vi "Spectrometer_R&S.vi"(11 "position_xyz":T2 {"Position Z" min=0.0 max=10.0 step=0.001 format="%.3f"; "Position Y" min=-10.0 max=10.0 step=0.1 format="%.3f"; "Position X" min=-10.0 max=10.0 step=0.1 format="%.3f"}) -> ()   [LabVIEW 2014]
uses:
  <vilib>/DAQmx/write.llb/DAQmx Write (Digital Bool 1Line 1Point).vi
  <vilib>/Analysis/baseanly.llb/Vector x A.vi
  GLOBAL_VAR.vi
  <vilib>/DAQmx/miscellaneous.llb/DAQmx Fill In Error Info.vi
  <vilib>/Analysis/Matrix/Numeric/Conversions/Array To Matrix - RA2.vi
  <vilib>/DAQmx/create/channels.llb/DAQmx Create Channel (CO-Pulse Generation-Ticks).vi
  <vilib>/DAQmx/create/channels.llb/DAQmx Create Channel (DO-Digital Output).vi
  <vilib>/DAQmx/configure/trigger.llb/DAQmx Start Trigger (Digital Edge).vi
  <resource>/objmgr/daqmx.rc
  <vilib>/Analysis/NI_AALBase.lvlib
  <vilib>/Analysis/Matrix/NI_Matrix.lvlib
  <instrlib>/Rohde&Schwarz RF Signal Generator/Rohde&Schwarz RF Signal Generator.lvlib
panel:
  in  "sweep_parameters":T1={"Repetitions"=1, "Power dBm"=5.999999061226845, "Freq Start [Hz]"=2800000000.0, "Freq Stop [Hz]"=3000000000.0, "Step size [Hz]"=2500000.0, "Dwell Time [ms]"=0.09999999974525053} {"Dwell Time [ms]" min=9.999999747378752e-05 max=4290.0 step=9.999999974752427e-07 format="%.3f"; "Step size [Hz]" min=10000.0 max=20000000000.0 step=1.0 format="%.2p"; "Freq Stop [Hz]" min=10000.0 max=20000000000.0 step=10000.0 format="%.2p"; "Freq Start [Hz]" min=10000.0 max=20000000000.0 step=10000.0 format="%.2p"; "Power dBm" min=-36.0 max=27.0 step=0.009999999776482582 format="%.2f"; "Repetitions" min=1 max=1000 step=1}
  out "File name":string
  in  "Save":bool
  in  "Stop":bool
  out "Run":i32=100
  out "Remain":i32
  out "Intensity Graph":ext[][](graph)
  out "Histogram":cluster{ext[], ext[]}[](graph)=[{[2700000000.0, 2702500000.0, 2705000000.0, 2707500000.0, 2710000000.0, 2712500000.0, 2715000000.0, 2717500000.0, 2720000000.0, 2722500000.0, 2725000000.0, 2727500000.0, 2730000000.0, 2732500000.0, 2735000000.0, 2737500000.0, 2740000000.0, 2742500000.0, 2745000000.0, 2747500000.0, 2750000000.0, 2752500000.0, 2755000000.0, 2757500000.0, 2760000000.0, 2762500000.0, 2765000000.0, 2767500000.0, 2770000000.0, 2772500000.0, 2775000000.0, 2777500000.0, 2780000000.0, 2782500000.0, 2785000000.0, 2787500000.0, 2790000000.0, 2792500000.0, 2795000000.0, 2797500000.0, 2800000000.0, 2802500000.0, 2805000000.0, 2807500000.0, 2810000000.0, 2812500000.0, 2815000000.0, 2817500000.0, 2820000000.0, 2822500000.0, 2825000000.0, 2827500000.0, 2830000000.0, 2832500000.0, 2835000000.0, 2837500000.0, 2840000000.0, 2842500000.0, 2845000000.0, 2847500000.0, 2850000000.0, 2852500000.0, 2855000000.0, 2857500000.0, 2860000000.0, 2862500000.0, 2865000000.0, 2867500000.0, 2870000000.0, 2872500000.0, 2875000000.0, 2877500000.0, 2880000000.0, 2882500000.0, 2885000000.0, 2887500000.0, 2890000000.0, 2892500000.0, 2895000000.0, 2897500000.0, 2900000000.0, 2902500000.0, 2905000000.0, 2907500000.0, 2910000000.0, 2912500000.0, 2915000000.0, 2917500000.0, 2920000000.0, 2922500000.0, 2925000000.0, 2927500000.0, 2930000000.0, 2932500000.0, 2935000000.0, 2937500000.0, 2940000000.0, 2942500000.0, 2945000000.0, 2947500000.0, 2950000000.0, 2952500000.0, 2955000000.0, 2957500000.0, 2960000000.0, 2962500000.0, 2965000000.0, 2967500000.0, 2970000000.0, 2972500000.0, 2975000000.0, 2977500000.0, 2980000000.0, 2982500000.0, 2985000000.0, 2987500000.0, 2990000000.0, 2992500000.0, 2995000000.0, 2997500000.0, 3000000000.0], [26841.121559672197128, 27464.174520667373477, 27576.32405364650522, 29408.099758972323686, 27638.629349746022854, 27576.32405364650522, 27638.629349746022854, 27651.09040896592638, 28398.753962160138, 28311.526547620813311, 28236.76019230139215, 27912.772652583900449, 27850.467356484382814, 27875.389474924189868, 28174.454896201874515, 28697.819383437822648, 28685.35832421791912, 28535.825613579076798, 28809.968916416954391, 29046.729041595121403, 28647.975146558208541, 28523.36455435917327, 28062.305363222742772, 28174.454896201874515, 28473.520317479559163, 27738.31782350525107, 28423.676080599945054, 29133.956456134446093, 28859.8131532965685, 27638.629349746022854, 29133.956456134446093, 27763.239941945058124, 27352.024987688241733, 27439.252402227566423, 28822.429975636857918, 27526.479816766891112, 28548.286672798980325, 27838.006297264479286, 28847.352094076664972, 28884.735271736375553, 29271.02810755338489, 28884.735271736375553, 27289.7196915887241, 28971.962686275700243, 28336.448666060620365, 28548.286672798980325, 27975.077948683418082, 27763.239941945058124, 29470.405055071841321, 28822.429975636857918, 28087.227481662549826, 28286.604429181006259, 27352.024987688241733, 27401.869224567855841, 28398.753962160138, 29308.411285213095471, 28485.98137669946269, 28585.669850458690906, 28710.280442657726175, 28236.76019230139215, 28311.526547620813311, 27576.32405364650522, 27302.180750808627625, 28299.065488400909786, 26878.504737331907709, 28809.968916416954391, 29420.560818192227213, 28859.8131532965685, 27750.778882725154597, 28535.825613579076798, 28398.753962160138, 28261.682310741199204, 28947.040567835893189, 28361.370784500427419, 28785.046797977147337, 28610.59196889849796, 27476.635579887277004, 28062.305363222742772, 28311.526547620813311, 28809.968916416954391, 28647.975146558208541, 28112.14960010235688, 28822.429975636857918, 27738.31782350525107, 28199.377014641681569, 28510.903495139269744, 27451.71346144746995, 28074.766422442646299, 27725.856764285347543, 28635.514087338305014, 28834.891034856761445, 27376.947106128048787, 29096.573278474735512, 28274.143369961102731, 29034.267982375217876, 28560.747732018883852, 27277.258632368820573, 28884.735271736375553, 28049.844304002839245, 27975.077948683418082, 26965.732151871232396, 28809.968916416954391, 28000.000067123225136, 27127.725921729978248, 28037.383244782935718, 28000.000067123225136, 27277.258632368820573, 27800.623119604768705, 28087.227481662549826, 27501.557698327084058, 26778.816263572679492, 26429.906605415380737, 27526.479816766891112, 26442.367664635284264, 26479.750842294994845, 27775.701001164961651, 27040.498507190653559, 26429.906605415380737, 27750.778882725154597, 27464.174520667373477, 27925.233711803803976]}, {[2700000000.0, 2702500000.0, 2705000000.0, 2707500000.0, 2710000000.0, 2712500000.0, 2715000000.0, 2717500000.0, 2720000000.0, 2722500000.0, 2725000000.0, 2727500000.0, 2730000000.0, 2732500000.0, 2735000000.0, 2737500000.0, 2740000000.0, 2742500000.0, 2745000000.0, 2747500000.0, 2750000000.0, 2752500000.0, 2755000000.0, 2757500000.0, 2760000000.0, 2762500000.0, 2765000000.0, 2767500000.0, 2770000000.0, 2772500000.0, 2775000000.0, 2777500000.0, 2780000000.0, 2782500000.0, 2785000000.0, 2787500000.0, 2790000000.0, 2792500000.0, 2795000000.0, 2797500000.0, 2800000000.0, 2802500000.0, 2805000000.0, 2807500000.0, 2810000000.0, 2812500000.0, 2815000000.0, 2817500000.0, 2820000000.0, 2822500000.0, 2825000000.0, 2827500000.0, 2830000000.0, 2832500000.0, 2835000000.0, 2837500000.0, 2840000000.0, 2842500000.0, 2845000000.0, 2847500000.0, 2850000000.0, 2852500000.0, 2855000000.0, 2857500000.0, 2860000000.0, 2862500000.0, 2865000000.0, 2867500000.0, 2870000000.0, 2872500000.0, 2875000000.0, 2877500000.0, 2880000000.0, 2882500000.0, 2885000000.0, 2887500000.0, 2890000000.0, 2892500000.0, 2895000000.0, 2897500000.0, 2900000000.0, 2902500000.0, 2905000000.0, 2907500000.0, 2910000000.0, 2912500000.0, 2915000000.0, 2917500000.0, 2920000000.0, 2922500000.0, 2925000000.0, 2927500000.0, 2930000000.0, 2932500000.0, 2935000000.0, 2937500000.0, 2940000000.0, 2942500000.0, 2945000000.0, 2947500000.0, 2950000000.0, 2952500000.0, 2955000000.0, 2957500000.0, 2960000000.0, 2962500000.0, 2965000000.0, 2967500000.0, 2970000000.0, 2972500000.0, 2975000000.0, 2977500000.0, 2980000000.0, 2982500000.0, 2985000000.0, 2987500000.0, 2990000000.0, 2992500000.0, 2995000000.0, 2997500000.0, 3000000000.0], [27662.305362263847, 27614.704116043806, 27558.75396014644, 27479.62623410005, 27635.264863756656, 27635.514084941045, 27523.73838373851, 27614.704116043802, 27583.17763621744, 27571.58885114293, 27593.520315369973, 27605.109100444486, 27505.545237277456, 27540.685424277577, 27573.831841802512, 27521.74461426332, 27747.788228512374, 27553.395704681883, 27408.099754177805, 27507.040564383846, 27553.769536458476, 27450.09352374888, 27547.16517507192, 27590.529661157172, 27485.98137430221, 27331.838071751987, 27460.06237112481, 27420.436202805507, 27402.99071989765, 27434.64181031619, 27576.697885423117, 27476.38635870286, 27470.654271461714, 27460.311592309215, 27451.962682631867, 27448.722807234688, 27469.781997316335, 27462.056140599987, 27364.23682572375, 27414.081062603364, 27456.573274543232, 27499.688539444087, 27488.598196738385, 27439.252402227583, 27451.215019078678, 27574.45489476352, 27513.894146954794, 27562.741499096825, 27559.377013107456, 27384.42374165998, 27576.074832462113, 27480.747729429848, 27504.423741947663, 27448.099754273695, 27508.90972326683, 27439.50162341197, 27397.383243248685, 27424.54835234809, 27331.21501879102, 27477.258632848276, 27459.68853934821, 27434.267978539607, 27381.05925567063, 27417.07171681613, 27347.912838145676, 27456.82249572762, 27392.398819560723, 27427.539006560855, 27402.86610930546, 27384.79757343659, 27482.86610949723, 27504.049910171063, 27508.037449121424, 27430.778881958024, 27495.202558124915, 27442.367667032533, 27426.16829004667, 27367.60131171313, 27402.616888121054, 27600.00006616432, 27539.68853953999, 27533.58262052224, 27462.305361784383, 27564.361436795392, 27572.087293511737, 27503.55146780227, 27476.137137518494, 27474.766421004293, 27580.560813781274, 27579.813150228085, 27592.024988263576, 27505.296016093063, 27570.84118758975, 27614.953337228195, 27611.215019462234, 27484.236826011424, 27503.925299578863, 27544.54835263575, 27602.616888600503, 27550.903492837893, 27593.769536554377, 27516.63557998317, 27611.962683015438, 27551.028103430108, 27655.701000877292, 27659.688539827646, 27578.5670443061, 27729.59508205134, 27610.093524132444, 27489.968913252564, 27615.202558412602, 27486.479816671, 27421.059255766515, 27418.56704392252, 27449.221249603488, 27600.996950901917, 27543.92529967475, 27425.17140530909, 27466.04367955036, 27523.987604922913, 27501.183866550484]}]
  in  "start":bool
  in  "stop":bool
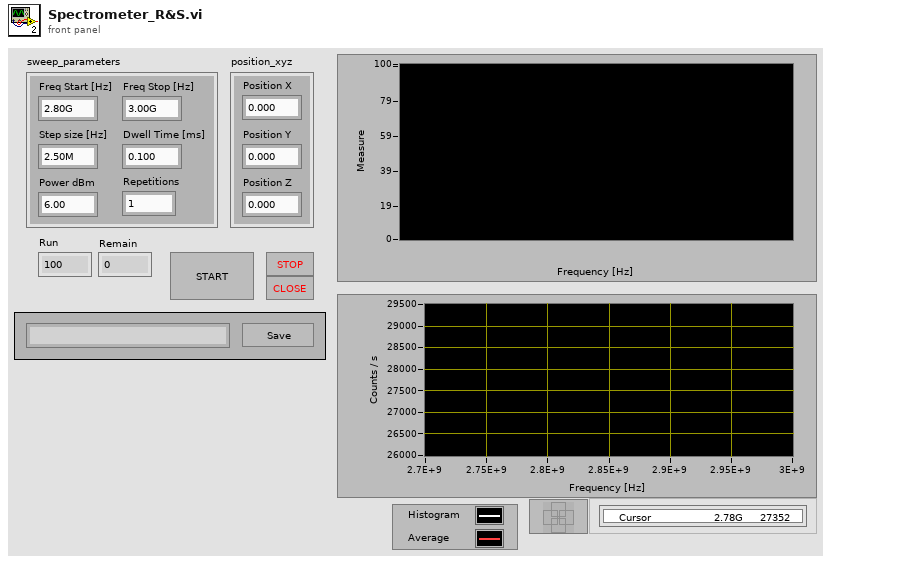
[diagram p1: front panel]
types:
  T1 = cluster{"Repetitions":i32, "Power dBm":dbl, "Freq Start [Hz]":dbl, "Freq Stop [Hz]":dbl, "Step size [Hz]":dbl, "Dwell Time [ms]":dbl}
  T2 = cluster{"Position X":dbl, "Position Y":dbl, "Position Z":dbl}
  T3 = enum16{"stand-by", "init", "config", "acquisition", "processing", "close", "Set Variables"}
  T4 = typedef "NI_Matrix.lvlib/RealMatrix.ctl" = dbl[][]
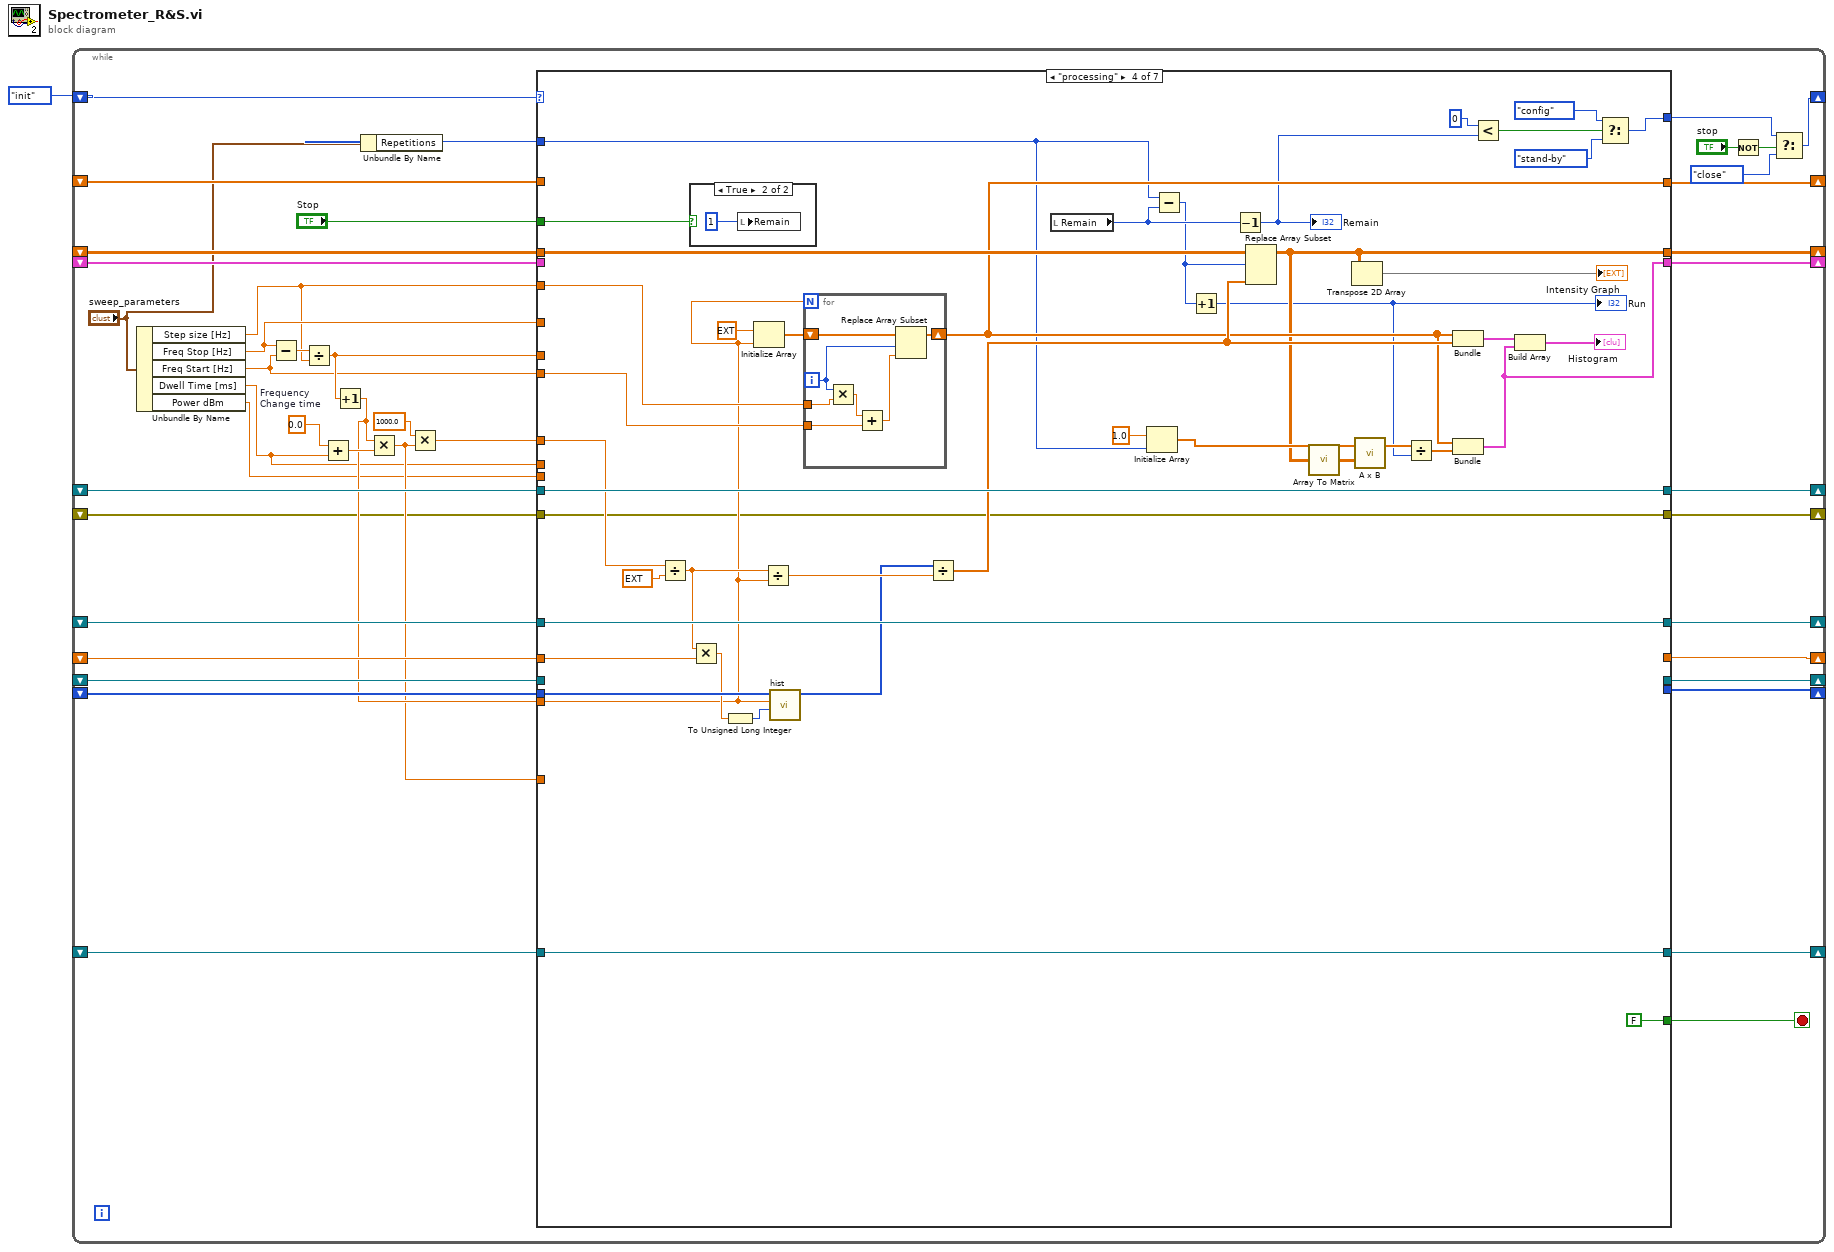
[diagram p0: block diagram]
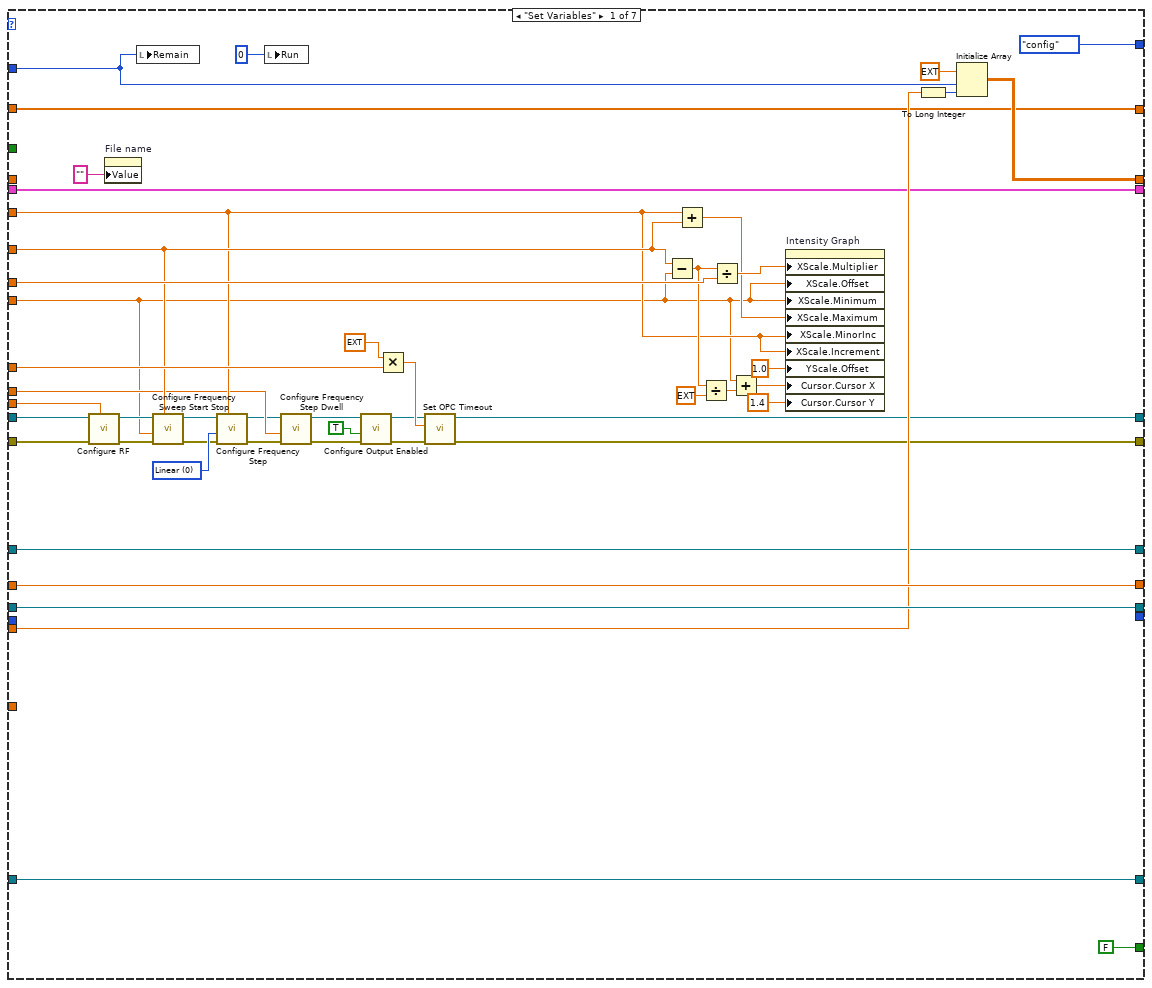
[diagram p2: hidden frame]
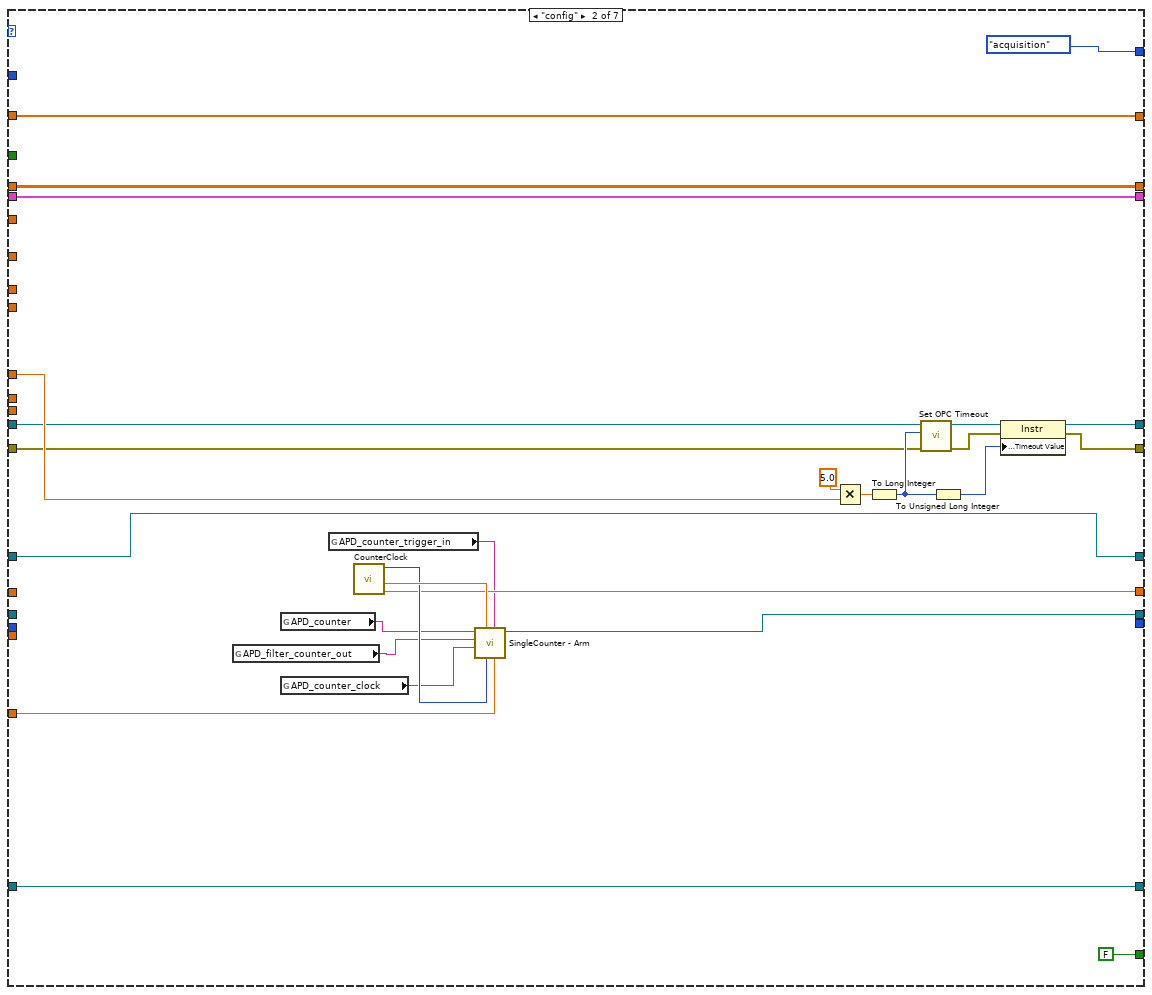
[diagram p3: hidden frame]
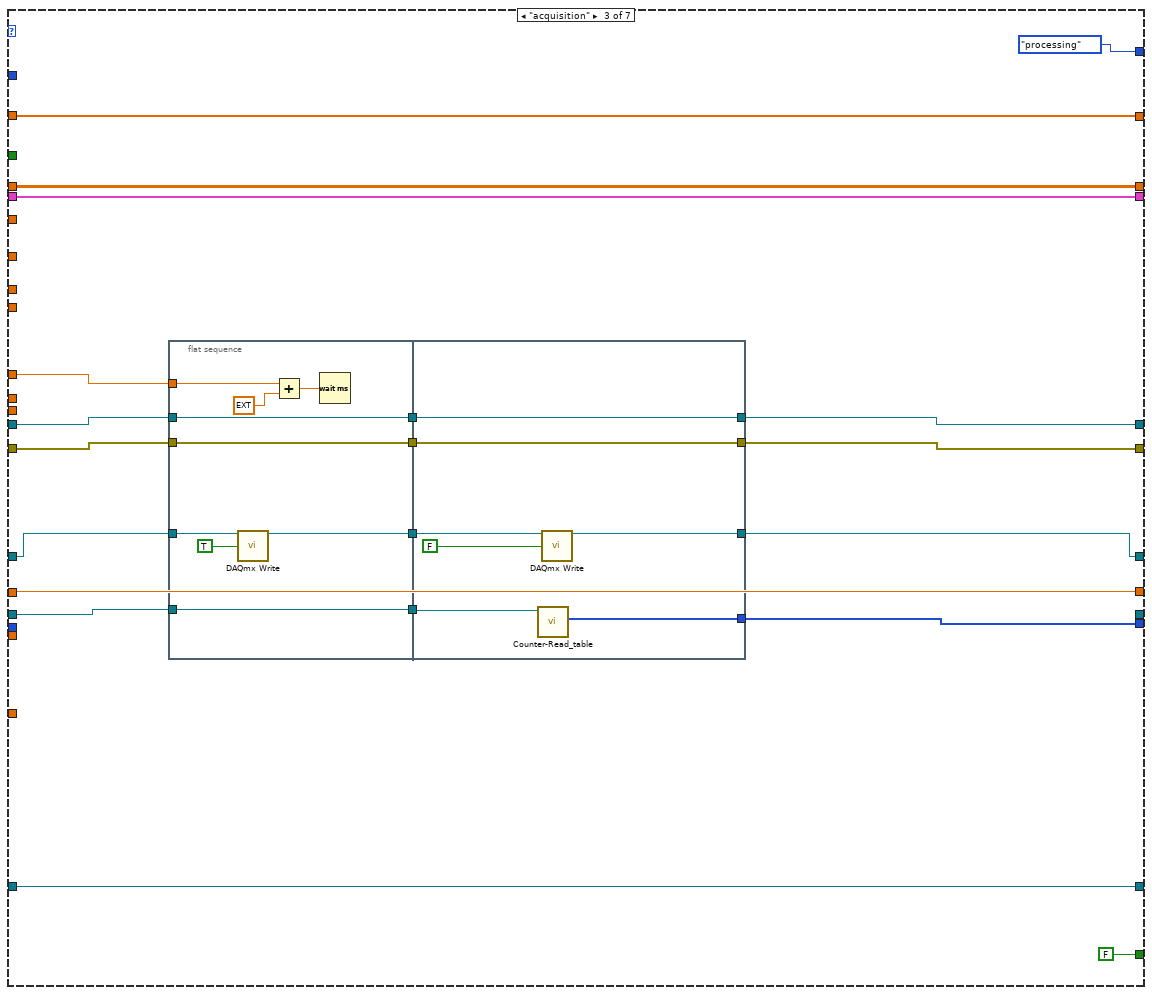
[diagram p4: hidden frame]
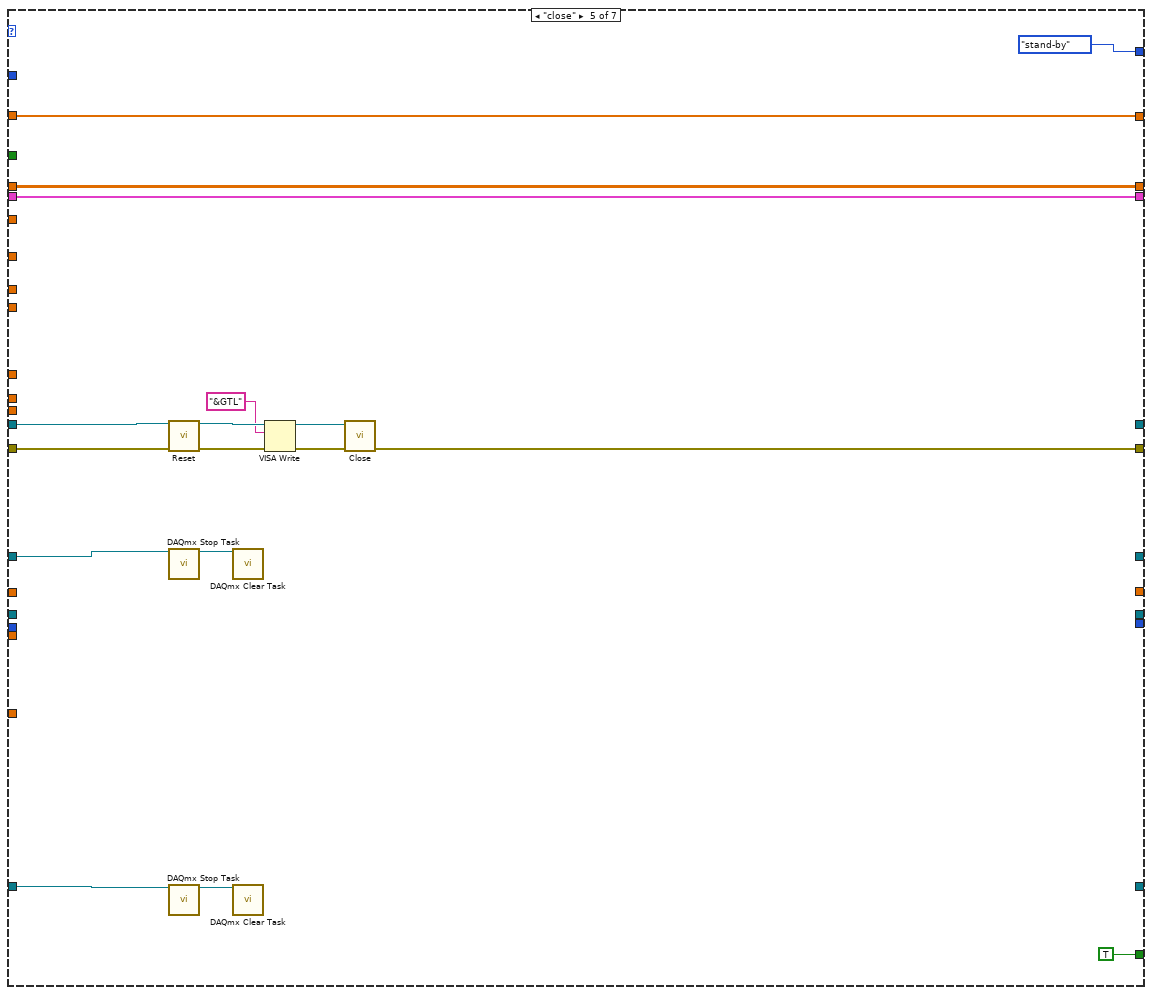
[diagram p6: hidden frame]
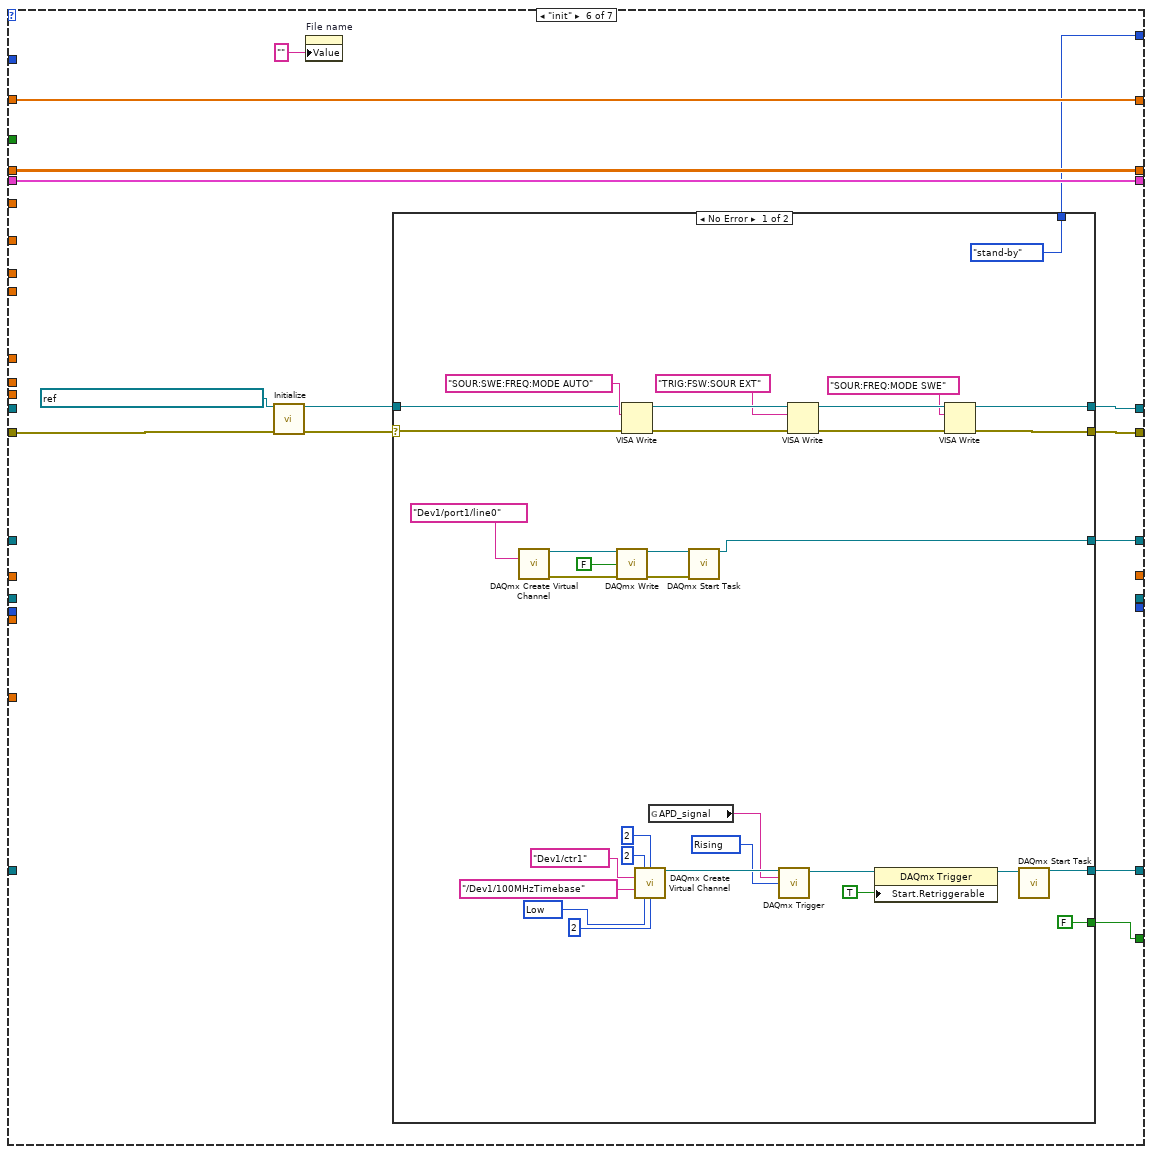
[diagram p7: hidden frame]
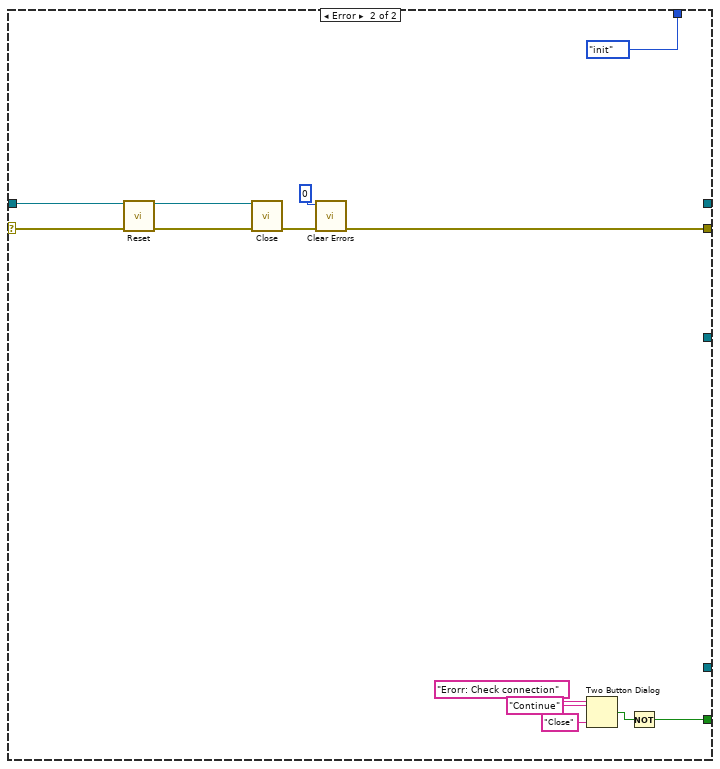
[diagram p8: hidden frame]
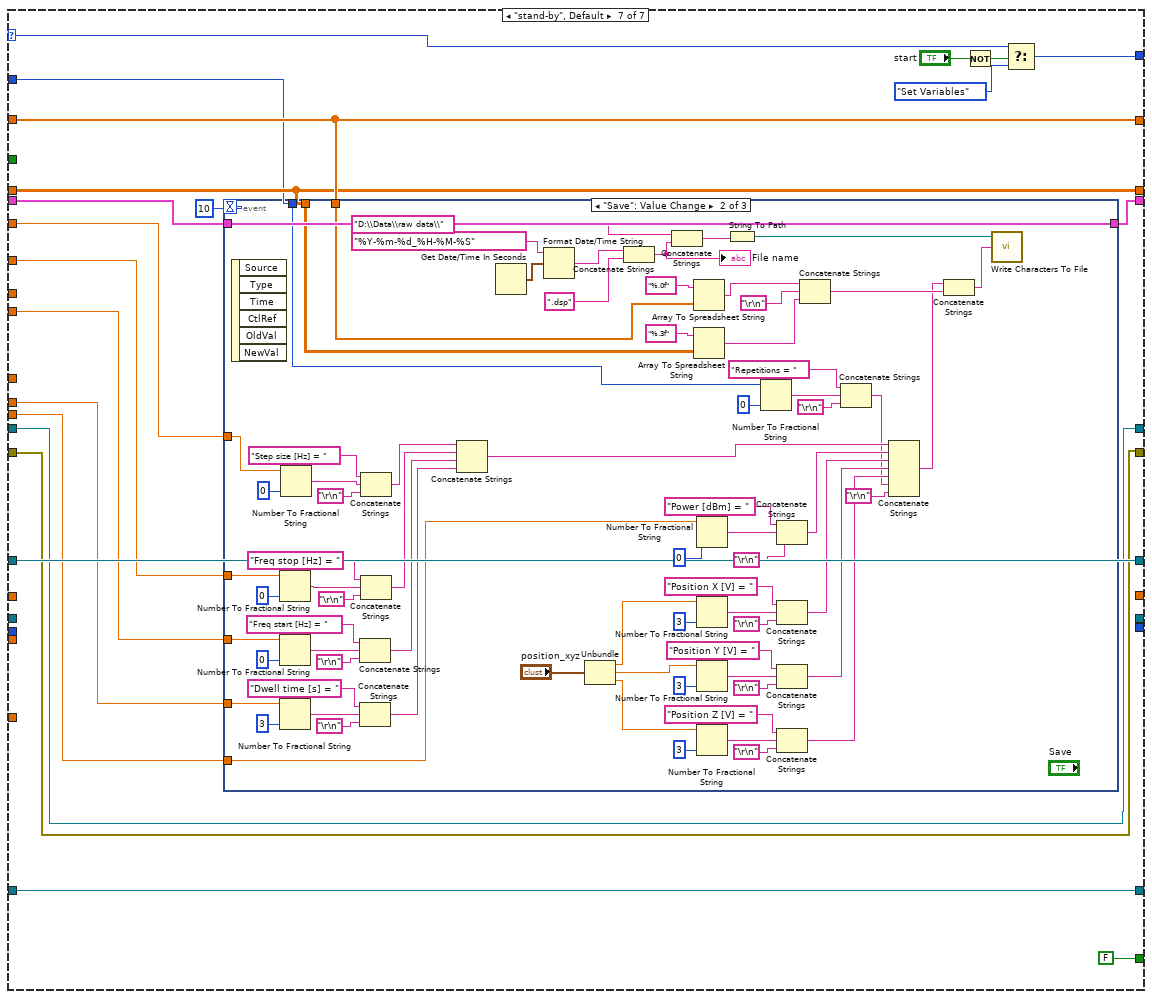
[diagram p9: hidden frame]
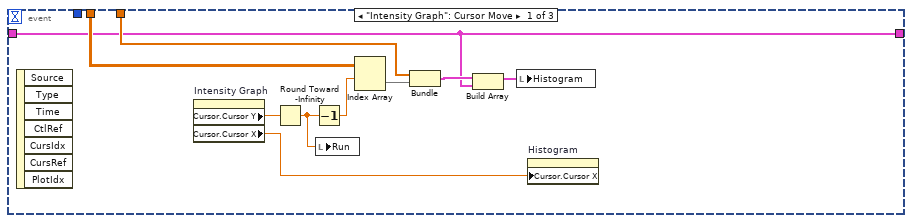
[diagram p10: hidden frame]
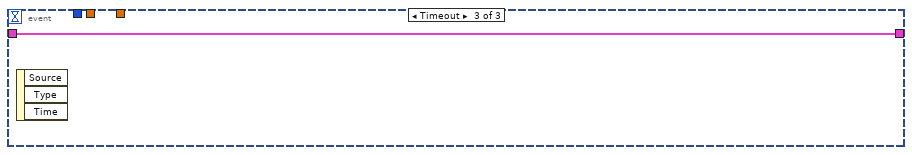
[diagram p11: hidden frame]
diagram:
  n1 = while {
    shift-right: [w30] -> _
    shift-left: T3."init" -> [w44]
    shift-right: [w40] -> _
    shift-left: _ -> [w39]
    shift-right: [w12] -> _
    shift-left: _ -> [w38]
    shift-right: [w37] -> _
    shift-left: _ -> [w36]
    shift-right: [w35] -> _
    shift-left: _ -> [w34]
    shift-right: [w28] -> _
    shift-left: _ -> [w27]
    shift-right: [w21] -> _
    shift-left: _ -> [w23]
    shift-right: [w20] -> _
    shift-left: _ -> [w19]
    shift-right: [w17] -> _
    shift-left: _ -> [w16]
    shift-right: [w15] -> _
    shift-left: _ -> [w14]
    shift-right: [w11] -> _
    shift-left: _ -> [w10]
    stop <- w29 stop-if-true
    w9 = 0.0  # Frequency Change time
    n2 = Unbundle By Name("sweep_parameters") -> ("Step size [Hz]"=w4:dbl, "Freq Stop [Hz]"=w5:dbl, "Freq Start [Hz]"=w3:dbl, "Dwell Time [ms]"=w6:dbl, "Power dBm"=w7:dbl)
    n3 = Subtract(x=w5, y=w3) -> (x-y=w43:dbl)
    n4 = Divide(x=w43, y=w4) -> (x/y=w24:dbl)
    n5 = Add(x=w9, y=w6) -> (x+y=w42:dbl)
    n6 = Increment(x=w24) -> (x+1=w25:dbl)
    n7 = Unbundle By Name("sweep_parameters") -> ("Repetitions"=w8:i32)
    n8 = Multiply(x=w25, y=w42) -> (x*y=w18:dbl)
    n9 = Multiply(x=1000.0 ("y"), y=w18) -> (x*y=w41:dbl)
    n10 = case shown="\"processing\"" w44 {
      selector: w44 -> [_ _ _ _ _ _ w304]
      tunnel: [T3."config" T3."acquisition" T3."processing" w184 T3."stand-by" w229 w303] -> w31
      tunnel: [w57 w104 w138 w192 _ w231 w284] -> w40
      tunnel: [w68 w119 w125 w191 _ w230 w301] -> w12
      tunnel: w39 -> [w55 w94 w139 w192 w220 _ w284]
      tunnel: w38 -> [w68 w119 w126 w191 w223 _ w301]
      tunnel: w4 -> [w64 _ _ w190 _ _ w291]
      tunnel: w5 -> [w66 _ _ _ _ _ w290]
      tunnel: w3 -> [w50 _ _ w178 _ _ w289]
      tunnel: w41 -> [w69 w107 w124 w187 _ _ _]
      tunnel: w6 -> [w63 _ _ _ _ _ w288]
      tunnel: [w88 w115 _ _ _ _ _] -> w37
      tunnel: w36 -> [w88 _ w137 _ _ _ _]
      tunnel: [_ _ w136 _ _ _ _] -> w35
      tunnel: w34 -> [_ _ _ w197 _ _ _]
      tunnel: [FALSE FALSE FALSE FALSE TRUE w227 FALSE] -> w29
      tunnel: [w87 w114 w134 _ _ _ _] -> w28
      tunnel: w27 -> [w87 _ w134 w195 _ _ _]
      tunnel: w25 -> [w84 _ _ w173 _ _ _]
      tunnel: w24 -> [w83 _ _ _ _ _ _]
      tunnel: w7 -> [w51 _ _ _ _ _ w287]
      tunnel: w8 -> [w74 _ _ w156 _ _ w286]
      tunnel: w23 -> [_ w113 w133 w181 w219 w237 w295]
      tunnel: [w86 w113 w133 w163 w219 w237 w295] -> w21
      tunnel: [w75 w111 w131 w169 w217 w236 w297] -> w20
      tunnel: w19 -> [w75 w111 w131 _ w217 w236 w297]
      tunnel: w18 -> [_ w110 _ _ _ _ _]
      tunnel: [w72 w109 w130 w175 _ w228 w294] -> w17
      tunnel: w16 -> [w72 w109 w130 w175 w215 _ w294]
      tunnel: [w71 w108 w129 w161 w214 w235 w292] -> w15
      tunnel: w14 -> [w71 w108 w129 _ w214 w235 w293]
      tunnel: "Stop" -> [_ _ _ w164 _ _ _]
      tunnel: [w56 w102 w127 w162 w212 w226 w285] -> w11
      tunnel: w10 -> [w54 w93 w128 w162 w213 w225 w285]
      frame "Set Variables" {
        w62 = 0 items=["Linear", "Logarithmic"] ("Scaling (Linear)")
        n11 = call <instrlib>:"Configure RF.vi"("Power Level (-30.0)"=w51, "error in (no error)"=w54, "VISA resource name"=w55) -> ("error out"=w53:errorcluster, "VISA resource name out"=w52:refnum<visa-resource-name>)  [unwired: 7 in]
        n12 = property on="File name" class="Str"("Value"="" ("File name")) -> ()  [unwired: 2 in, 2 out]
        n13 = local write "Remain"(w74) -> ()
        n14 = call <instrlib>:"Configure Frequency Sweep Start Stop.vi"("Stop (500.0e6)"=w66, "error in (no error)"=w53, "Start (100.0e6)"=w50, "VISA resource name"=w52) -> ("error out"=w60:errorcluster, "VISA resource name out"=w61:refnum<visa-resource-name>)  [unwired: 6 in]
        n15 = call <instrlib>:"Configure Frequency Step.vi"("Step Size (100.0e3)"=w64, "error in (no error)"=w60, "Scaling (Linear)"=w62, "VISA resource name"=w61) -> ("error out"=w58:errorcluster, "VISA resource name out"=w59:refnum<visa-resource-name>)  [unwired: 6 in]
        n16 = local write "Run"(0 ("Run")) -> ()
        n17 = call <instrlib>:"Configure Frequency Step Dwell.vi"("error in (no error)"=w58, "Dwell (10.0e-3)"=w63, "VISA resource name"=w59) -> ("error out"=w46:errorcluster, "VISA resource name out"=w48:refnum<visa-resource-name>)  [unwired: 7 in]
        n18 = call <instrlib>:"Configure Output Enabled.vi"("error in (no error)"=w46, "Output Enabled (Off)"=TRUE, "VISA resource name"=w48) -> ("error out"=w45:errorcluster, "VISA resource name out"=w47:refnum<visa-resource-name>)  [unwired: 7 in]
        n19 = Multiply(x=ext 1.100000023841858, y=w69) -> (x*y=w65:ext)
        n20 = call <instrlib>:"Set OPC Timeout.vi"("error in (no error)"=w45, "OPC Timeout (0)"=w65, "VISA resource name"=w47) -> ("error out"=w56:errorcluster, "VISA resource name out"=w57:refnum<visa-resource-name>)  [unwired: 7 in]
        n21 = Subtract(x=w66, y=w50) -> (x-y=w80:dbl)
        n22 = Add(x=w64, y=w66) -> (x+y=w82:dbl)
        n23 = Divide(x=w80, y=ext 2.0) -> (x/y=w76:ext)
        n24 = Divide(x=w80, y=w83) -> (x/y=w85:dbl)
        n25 = Add(x=w50, y=w76) -> (x+y=w77:ext)
        n26 = property on="Intensity Graph" class="IntGraph (strict)"("XScale.Multiplier"=w85, "XScale.Offset"=w50, "XScale.Minimum"=w50, "XScale.Maximum"=w82, "XScale.MinorInc"=w64, "XScale.Increment"=w64, "YScale.Offset"=1.0 ("Y Scale.Offset and Multiplier:Offset"), "Cursor.Cursor X"=w77, "Cursor.Cursor Y"=1.4 ("Cursor.Cursor Position:Cursor Y")) -> ()  [unwired: 2 in, 2 out]
        n27 = To Long Integer(number=w84) -> (32bit integer=w90:i32)
        n28 = Initialize Array(ext 0.0 ("element"), w74, w90) -> (w86:ext[][])
      }
      frame "config" {
        n29 = global read "GLOBAL_VAR.vi" "APD_filter_counter_out"() -> (w98:tag)
        n30 = global read "GLOBAL_VAR.vi" "APD_counter"() -> (w100:tag)
        n31 = global read "GLOBAL_VAR.vi" "APD_counter_clock"() -> (w99:tag)
        n32 = global read "GLOBAL_VAR.vi" "APD_counter_trigger_in"() -> (w101:tag)
        n33 = call "CounterClock.vi"() -> ("Counter clock rate divided by prescaler"=w114:dbl, "Counter clock rate"=w117:dbl, "CI.Prescaler"=w116:u32)  [unwired: 8 in, 1 out]
        n34 = call "SingleCounter - Arm.vi"("Duration"=w110, "Trigger Source"=w101, "CI.Prescaler"=w116, "Sampling Rate"=w117, "Clock Source"=w99, "External Timing Source"=w98, "counter"=w100) -> ("task out"=w115:refnum<k21>)  [unwired: 3 in, 1 out]
        n35 = Multiply(x=5.0 ("lower limit"), y=w107) -> (x*y=w97:dbl)
        n36 = To Long Integer(number=w97) -> (32bit integer=w96:i32)
        n37 = call <instrlib>:"Set OPC Timeout.vi"("error in (no error)"=w93, "OPC Timeout (0)"=w96, "VISA resource name"=w94) -> ("error out"=w103:errorcluster, "VISA resource name out"=w105:refnum<visa-resource-name>)  [unwired: 7 in]
        n38 = To Unsigned Long Integer(number=w96) -> (unsigned 32bit integer=w95:u32)
        n39 = property class="Instr"(reference=w105, error in=w103, "General Settings:Timeout Value"=w95) -> (reference out=w104:refnum<visa-resource-name>, error out=w102:errorcluster)
      }
      frame "acquisition" {
        n40 = flat-sequence {
          tunnel: w139 -> [w144]
          tunnel: [w147] -> w123
          tunnel: [w146] -> w122
          tunnel: w137 -> [w146]
          tunnel: w128 -> [w143]
          tunnel: w126 -> [w145]
          tunnel: w124 -> [w141]
          tunnel: [w144] -> w121
          tunnel: [w143] -> w120
          tunnel: [w151] -> w125
          tunnel: [w150] -> w138
          tunnel: w123 -> [w154]
          tunnel: w122 -> [w152]
          tunnel: [w153] -> w136
          tunnel: [w149] -> w127
          tunnel: w121 -> [w150]
          tunnel: w120 -> [w149]
          frame #0 {
            n41 = call-poly <vilib>:"DAQmx Write.vi"("task/channels in"=w145, "data"=TRUE) -> ("task out"=w147:refnum<k21>)  [unwired: 11 in, 2 out]
            n42 = Add(x=w141, y=ext 1.1) -> (x+y=w142:ext)
            n43 = Wait (ms)(milliseconds to wait=w142) -> ()  [unwired: 1 out]
          }
          frame #1 {
            n44 = call "Counter-Read_table.vi"("task in"=w152) -> ("time tags"=w153:u32[])  [unwired: 9 in, 1 out]
            n45 = call-poly <vilib>:"DAQmx Write.vi"("task/channels in"=w154, "data"=FALSE) -> ("task out"=w151:refnum<k21>)  [unwired: 11 in, 2 out]
          }
        }
      }
      frame "processing" {
        n46 = Divide(x=w187, y=ext 1000.0) -> (x/y=w186:ext)
        n47 = case shown="True" w164 {
          frame False {
          }
          frame True {
            n48 = local write "Remain"(1) -> ()
          }
        }
        n49 = Multiply(x=w186, y=w195) -> (x*y=w193:ext)
        n50 = To Unsigned Long Integer(number=w193) -> (unsigned 32bit integer=w194:u32)
        n51 = Initialize Array(ext 0.0 ("element"), w173) -> (w188:ext[])
        n52 = Divide(x=w186, y=w173) -> (x/y=w185:ext)
        n53 = call "hist.vi"("#clock cycles"=w194, "#bins"=w173, "counter timetag list"=w197) -> ("histogram"=w160:i32[])  [unwired: 7 in]
        n54 = for {
          N: w173 -> [_]
          tunnel: w190 -> [w202]
          shift-right: [w206] -> w169
          shift-left: w188 -> [w205]
          tunnel: w178 -> [w204]
          i -> [w203]
          n55 = Multiply(x=w203, y=w202) -> (x*y=w201:dbl)
          n56 = Add(x=w201, y=w204) -> (x+y=w200:dbl)
          n57 = Replace Array Subset(array=w205, new element=w200, index=w203) -> (w206:ext[])
        }
        n58 = Divide(x=w160, y=w185) -> (x/y=w174:ext[])
        n59 = local read "Remain"() -> (w177:i32)
        n60 = Initialize Array(1.0 ("element"), w156) -> (w170:dbl[])
        n61 = Subtract(x=w156, y=w177) -> (x-y=w176:i32)
        n62 = Increment(x=w176) -> (x+1=w158:i32)
        "Run" <- w158
        n63 = Decrement(x=w177) -> (x-1=w157:i32)
        "Remain" <- w157
        n64 = Replace Array Subset(array=w181, new element=w174, index (row)=w176) -> (w163:ext[][])  [unwired: 1 in]
        n65 = call-poly <vilib>:"Array To Matrix.vi"("Real 2D Array"=w163) -> ("Real Matrix"=w172:T4)
        n66 = Transpose 2D Array(2D array=w163) -> (transposed array=→"Intensity Graph":ext[][])
        n67 = call-poly <vilib>:"A x B.vi"("Matrix A"=w172, "Vector V'"=w170) -> ("V' x A"=w167:dbl[])  [unwired: 1 out]
        n68 = Divide(x=w167, y=w158) -> (x/y=w168:dbl[])
        n69 = Bundle(w169, w174) -> (w166:cluster{ext[], ext[]})  [unwired: 1 in]
        n70 = Bundle(w169, w168) -> (w161:cluster{ext[], dbl[]})  [unwired: 1 in]
        n71 = Less?(x=0, y=w157) -> (x < y?=w182:bool)
        n72 = Build Array(w166, w161) -> (→"Histogram":cluster{ext[], ext[]}[])
        n73 = Select(t=T3."config", s=w182, f=T3."stand-by") -> (s? t:f=w184:T3)
      }
      frame "close" {
        n74 = call <instrlib>:"Reset.vi"("VISA resource name"=w220, "error in (no error)"=w213) -> ("VISA resource name out"=w211:refnum<visa-resource-name>, "error out"=w209:errorcluster)  [unwired: 12 in]
        n75 = call <vilib>:"DAQmx Stop Task.vi"("task/channels in"=w223) -> ("task out"=w222:refnum<k21>)  [unwired: 13 in, 1 out]
        n76 = call <vilib>:"DAQmx Stop Task.vi"("task/channels in"=w215) -> ("task out"=w216:refnum<k21>)  [unwired: 13 in, 1 out]
        n77 = call <vilib>:"DAQmx Clear Task.vi"("task in"=w222) -> ()  [unwired: 14 in, 1 out]
        n78 = call <vilib>:"DAQmx Clear Task.vi"("task in"=w216) -> ()  [unwired: 14 in, 1 out]
        n79 = VISA Write(VISA resource name=w211, write buffer="&GTL", error in (no error)=w209) -> (VISA resource name out=w210:refnum<visa-resource-name>, error out=w208:errorcluster)  [unwired: 1 out]
        n80 = call <instrlib>:"Close.vi"("error in (no error)"=w208, "VISA resource name"=w210) -> ("error out"=w212:errorcluster)  [unwired: 9 in]
      }
      frame "init" {
        n81 = call <instrlib>:"Initialize.vi"("VISA resource name"=refnum<visa-resource-name> "USB0::0x0AAD::0x005F::262159::INSTR", "error in (no error)"=w225) -> ("VISA resource name out"=w232:refnum<visa-resource-name>, "error out"=w233:errorcluster)  [unwired: 12 in]
        n82 = property on="File name" class="Str"("Value"="" ("File name")) -> ()  [unwired: 2 in, 2 out]
        n83 = case shown="No Error" w233 {
          selector: w233 -> [w249 w282]
          tunnel: [w247 _] -> w231
          tunnel: w232 -> [w246 w283]
          tunnel: [w239 _] -> w230
          tunnel: [T3."stand-by" T3."init"] -> w229
          tunnel: [w258 _] -> w228
          tunnel: [FALSE w274] -> w227
          tunnel: [w248 w271] -> w226
          frame No Error {
            w264 = 10280 items=["Rising"=10280, "Falling"=10171] ("edge")
            w260 = 10214 items=["High"=10192, "Low"=10214] ("idle state")
            n84 = call-poly <vilib>:"DAQmx Create Virtual Channel.vi"("lines"=tag "Dev1/port1/line0") -> ("task out"=w240:refnum<k21>, "error out"=w243:errorcluster)  [unwired: 13 in]
            n85 = call-poly <vilib>:"DAQmx Write.vi"("task/channels in"=w240, "data"=FALSE, "error in"=w243) -> ("task out"=w242:refnum<k21>, "error out"=w244:errorcluster)  [unwired: 10 in, 1 out]
            n86 = VISA Write(VISA resource name=w246, write buffer="SOUR:SWE:FREQ:MODE AUTO", error in (no error)=w249) -> (VISA resource name out=w256:refnum<visa-resource-name>, error out=w253:errorcluster)  [unwired: 1 out]
            n87 = call-poly <vilib>:"DAQmx Create Virtual Channel.vi"("high ticks"=u32 2, "low ticks"=u32 2, "counter"=tag "Dev1/ctr1", "source of ticks"=tag "/Dev1/100MHzTimebase", "idle state"=w260, "initial delay"=u32 2) -> ("task out"=w269:refnum<k21>)  [unwired: 8 in, 1 out]
            n88 = global read "GLOBAL_VAR.vi" "APD_signal"() -> (w238:tag)
            n89 = call <vilib>:"DAQmx Start Task.vi"("task/channels in"=w242, "error in"=w244) -> ("task out"=w239:refnum<k21>)  [unwired: 12 in, 1 out]
            n90 = call-poly <vilib>:"DAQmx Trigger.vi"("task/channels in"=w269, "source"=w238, "edge"=w264) -> ("task out"=w265:refnum<k21>)  [unwired: 11 in, 1 out]
            n91 = VISA Write(VISA resource name=w256, write buffer="TRIG:FSW:SOUR EXT" ("write buffer 2"), error in (no error)=w253) -> (VISA resource name out=w255:refnum<visa-resource-name>, error out=w254:errorcluster)  [unwired: 1 out]
            n92 = property class="DAQmx Trigger"(reference=w265, "Start.Retriggerable"=TRUE) -> (reference out=w267:refnum<k21>)  [unwired: 1 in, 1 out]
            n93 = VISA Write(VISA resource name=w255, write buffer="SOUR:FREQ:MODE SWE" ("write buffer 3"), error in (no error)=w254) -> (VISA resource name out=w247:refnum<visa-resource-name>, error out=w248:errorcluster)  [unwired: 1 out]
            n94 = call <vilib>:"DAQmx Start Task.vi"("task/channels in"=w267) -> ("task out"=w258:refnum<k21>)  [unwired: 13 in, 1 out]
          }
          frame Error {
            n95 = call <instrlib>:"Reset.vi"("VISA resource name"=w283, "error in (no error)"=w282) -> ("VISA resource name out"=w273:refnum<visa-resource-name>, "error out"=w272:errorcluster)  [unwired: 12 in]
            n96 = call <instrlib>:"Close.vi"("error in (no error)"=w272, "VISA resource name"=w273) -> ("error out"=w278:errorcluster)  [unwired: 9 in]
            n97 = call <vilib>:"Clear Errors.vi"("error in (no error)"=w278, "specific error code to clear (0: all)"=0) -> ("error out"=w271:errorcluster)  [unwired: 4 in, 1 out]
            n98 = Two Button Dialog(message="Erorr: Check connection", 1:"Close" ("F button name (\"Cancel\")"), 2:"Continue" ("T button name (\"OK\")")) -> (T button?=w275:bool)
            n99 = Not(x=w275) -> (.not. x?=w274:bool)
          }
        }
      }
      frame "stand-by", Default {
        n100 = event shown="[1] \"Save\": Value Change" {
          selector: _ -> [_ _ _]
          dyn-events: _ -> [_ _ _]
          timeout: 10 -> [_ _ _]
          tunnel: w297 -> [w314 w381 _]
          tunnel: w295 -> [w310 w384 _]
          tunnel: w293 -> [w305 w385 w391]
          tunnel: [w305 w385 w391] -> w292
          tunnel: w291 -> [_ w369 _]
          tunnel: w290 -> [_ w366 _]
          tunnel: w289 -> [_ w363 _]
          tunnel: w288 -> [_ w358 _]
          tunnel: w287 -> [_ w353 _]
          tunnel: w286 -> [_ w336 _]
          event "Intensity Graph": Cursor Move {
            n101 = event-data() -> ()  [unwired: 1 in, 7 out]
            n102 = property on="Intensity Graph" class="IntGraph (strict)"() -> ("Cursor.Cursor Y"=w312:dbl, "Cursor.Cursor X"=w308:dbl)  [unwired: 2 in, 2 out]
            n103 = Round Toward -Infinity(1:w312) -> (0:w309:dbl)
            n104 = Decrement(x=w309) -> (x-1=w311:dbl)
            n105 = local write "Run"(w309) -> ()
            n106 = Index Array(array=w310, index (row)=w311) -> (element=w313:ext[])  [unwired: 1 in]
            n107 = Bundle(w314, w313) -> (w306:cluster{ext[], ext[]})  [unwired: 1 in]
            n108 = Build Array(w306, w305) -> (w307:cluster{ext[], ext[]}[])
            n109 = local write "Histogram"(w307) -> ()
            n110 = property on="Histogram" class="XYGraph (strict)"("Cursor.Cursor X"=w308) -> ()  [unwired: 2 in, 2 out]
          }
          event "Save": Value Change {
            n111 = event-data() -> ()  [unwired: 1 in, 6 out]
            n112 = Number To Fractional String(number=w366, precision (6)=i16 0) -> (F-format string=w367:string)  [unwired: 2 in]
            n113 = Number To Fractional String(number=w363, precision (6)=i16 0) -> (F-format string=w364:string)  [unwired: 2 in]
            n114 = Number To Fractional String(number=w358, precision (6)=i16 3) -> (F-format string=w360:string)  [unwired: 2 in]
            n115 = Number To Fractional String(number=w369, precision (6)=i16 0) -> (F-format string=w370:string)  [unwired: 2 in]
            n116 = Concatenate Strings("Freq start [Hz] = ", w364, "\r\n") -> (w333:string)
            n117 = Concatenate Strings("Dwell time [s] = ", w360, "\r\n") -> (w332:string)
            n118 = Concatenate Strings("Step size [Hz] = ", w370, "\r\n") -> (w335:string)
            n119 = Concatenate Strings("Freq stop [Hz] = ", w367, "\r\n") -> (w334:string)
            n120 = Concatenate Strings(w335, w334, w333, w332) -> (w328:string)
            n121 = Get Date/Time In Seconds() -> (seconds since 1Jan1904=w390:timestamp)
            n122 = Format Date/Time String(time format string (%c)="%Y-%m-%d_%H-%M-%S", seconds (now)=w390) -> (date/time string=w389:string)  [unwired: 1 in]
            n123 = Unbundle("position_xyz") -> ("Position X"=w317:dbl, "Position Y"=w316:dbl, "Position Z"=w315:dbl)
            n124 = Concatenate Strings(w389, ".dsp") -> (w321:string)
            "File name" <- w321
            n125 = Concatenate Strings("D:\\Data\\raw data\\", w321) -> (w319:string)
            n126 = Array To Spreadsheet String(array=w381, 3:"%.0f" ("format string")) -> (spreadsheet string=w380:string)  [unwired: 1 in]
            n127 = Array To Spreadsheet String(array=w384, 3:"%.3f" ("format string")) -> (spreadsheet string=w378:string)  [unwired: 1 in]
            n128 = Number To Fractional String(number=w353, precision (6)=i16 0) -> (F-format string=w355:string)  [unwired: 2 in]
            n129 = Number To Fractional String(number=w317, precision (6)=i16 3) -> (F-format string=w347:string)  [unwired: 2 in]
            n130 = Number To Fractional String(number=w316, precision (6)=i16 3) -> (F-format string=w344:string)  [unwired: 2 in]
            n131 = Number To Fractional String(number=w315, precision (6)=i16 3) -> (F-format string=w338:string)  [unwired: 2 in]
            n132 = String To Path(string=w319) -> (path=w386:path)
            n133 = Number To Fractional String(number=w336, precision (6)=i16 0) -> (F-format string=w352:string)  [unwired: 2 in]
            n134 = Concatenate Strings("Power [dBm] = ", w355, "\r\n") -> (w327:string)
            n135 = Concatenate Strings("Position X [V] = ", w347, "\r\n") -> (w326:string)
            n136 = Concatenate Strings("Position Y [V] = ", w344, "\r\n") -> (w325:string)
            n137 = Concatenate Strings("Position Z [V] = ", w338, "\r\n") -> (w324:string)
            n138 = Concatenate Strings(w380, "\r\n", w378) -> (w330:string)
            n139 = Concatenate Strings("Repetitions = ", w352, "\r\n") -> (w323:string)
            n140 = Concatenate Strings(w328, w327, w326, w325, w324, w323, "\r\n") -> (w329:string)
            n141 = Concatenate Strings(w329, w330) -> (w331:string)
            n142 = call <vilib>:"Write Characters To File.vi"("character string"=w331, "file path (dialog if empty)"=w386) -> ()  [unwired: 3 in, 1 out]
          }
          event Timeout {
            n143 = event-data() -> ()  [unwired: 1 in, 3 out]
          }
        }
        n144 = Not(x="start") -> (.not. x?=w302:bool)
        n145 = Select(t=w304, s=w302, f=T3."Set Variables") -> (s? t:f=w303:T3)
      }
    }
    n146 = Not(x="stop") -> (.not. x?=w33:bool)
    n147 = Select(t=w31, s=w33, f=T3."close") -> (s? t:f=w30:T3)
  }
